vi "_Get Interfaces.vi"(8 "error in (no error)":errorcluster, 11 "Numeric in":refnum<class "Numeric Test Object.lvclass">) -> (0 "error out":errorcluster, 2 "Concrete Interfaces":refnum<class "IUnknown.lvclass">[](array[class]), 3 "Numeric out":refnum<class "Numeric Test Object.lvclass">)   [LabVIEW 2009, in "Numeric Test Object.lvclass"]
doc: "Returns an array of all the concrete interfaces implemented for the given interfaceable object. Child classes must override this vi."
uses:
  Numeric Test Object.lvclass
  Source/IUnknown Class/IUnknown.lvclass
  Interface Implementations/IIntByVal/IIntByVal.lvclass
  Interface Implementations/IIntByRef (DVR)/IIntByRef (DVR).lvclass
  Interface Implementations/IIntByRef (Unnamed SEQ)/IIntByRef (Unnamed SEQ).lvclass
  Interface Implementations/IIntStatic (Global)/IIntStatic (Global).lvclass
  Interface Implementations/IIntStatic (Named SEQ)/IIntStatic (Named SEQ).lvclass
  Interface Implementations/IIntStatic (Func Global)/IIntStatic (Func Global).lvclass
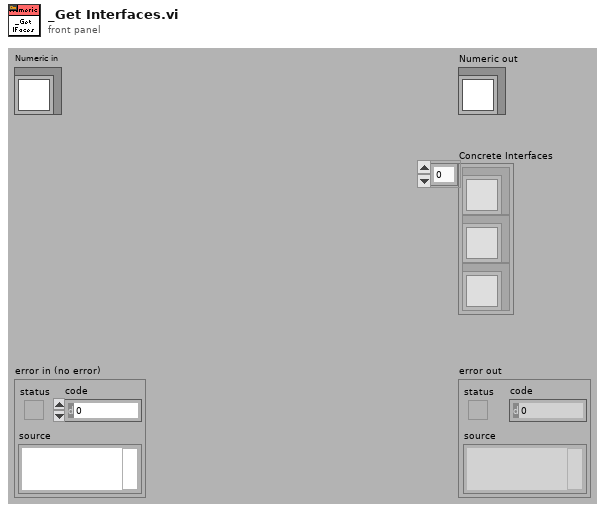
[diagram p1: front panel]
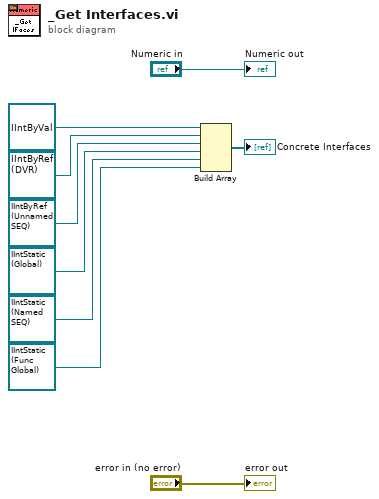
[diagram p0: block diagram]
diagram:
  n1 = Build Array(refnum<class "IIntByVal.lvclass"> refnum ("IIntByVal.lvclass"), refnum<class "IIntByRef (DVR).lvclass"> refnum ("IIntByRef.lvclass"), refnum<class "IIntByRef (Unnamed SEQ).lvclass"> refnum ("IIntByRef (Unnamed SEQ)"), refnum<class "IIntStatic (Global).lvclass"> refnum ("IIntStatic (Global).lvclass"), refnum<class "IIntStatic (Named SEQ).lvclass"> refnum ("IIntStatic"), refnum<class "IIntStatic (Func Global).lvclass"> refnum ("IIntStatic 2")) -> (→"Concrete Interfaces":refnum<class "IInt.lvclass">[])
  "error out" <- "error in (no error)"
  "Numeric out" <- "Numeric in"
